vi "DIAdem Stop.vi"(5 "error in (no error)":errorcluster, 8 "DIAdem Reference":T1) -> (0 "error out":errorcluster)   [LabVIEW 2011]
uses:
  <vilib>/ExportToExcel/DIAdem Reference.ctl
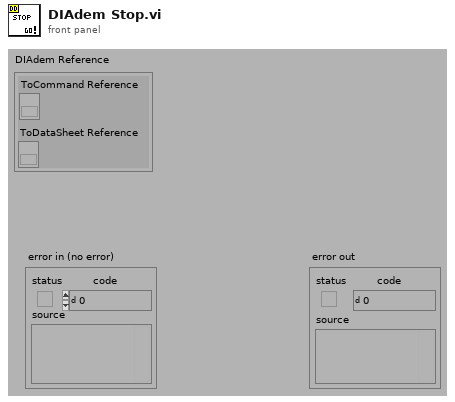
[diagram p1: front panel]
types:
  T1 = typedef "DIAdem Reference.ctl" = cluster{"ToCommand Reference":refnum<k7>, "ToDataSheet Reference":refnum<k7>}
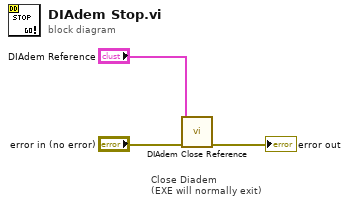
[diagram p0: block diagram]
diagram:
  # "Close Diadem\n(EXE will normally exit)"
  n1 = call <vilib>:"DIAdem Close Reference.vi"("error in (no error)"="error in (no error)", "DIAdem Reference"="DIAdem Reference") -> ("error out"=→"error out":errorcluster)  [unwired: 9 out]
